vi "Reset All CMDS.vi"(8 "error in (no error)":errorcluster) -> (0 "error out":errorcluster)   [LabVIEW 2018]
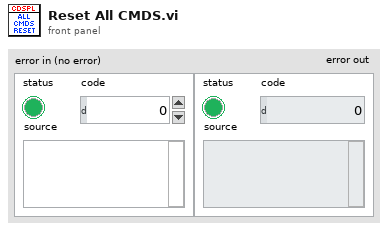
[diagram p1: front panel]
types:
  T1 = enum16{"Lamp A1", "Lamp B1", "Lamp C1", "Lamp D1", "Lamp E1", "Lamp F1", "Lamp G1", "Lamp H1", "Lamp A2", "Lamp B2", "Lamp C2", "Lamp D2", "Lamp E2", "Lamp F2", "Lamp G2", "Lamp H2", "Ack A1", "Ack B1", "Ack C1", "Ack D1", "Ack E1", "Ack F1", "Ack G1", "Ack H1", "Ack A2", "Ack B2", "Ack C2", "Ack D2", "Ack E2", "Ack F2", "Ack G2", "Ack H2", "SSM", "SAS", "LSM", ""}
  T2 = enum16{"Lamp A1", "Lamp B1", "Lamp C1", "Lamp D1", "Lamp E1", "Lamp F1", "Lamp G1", "Lamp H1", "Lamp A2", "Lamp B2", "Lamp C2", "Lamp D2", "Lamp E2", "Lamp F2", "Lamp G2", "Lamp H2", "Ack A1", "Ack B1", "Ack C1", "Ack D1", "Ack E1", "Ack F1", "Ack G1", "Ack H1", "Ack A2", "Ack B2", "Ack C2", "Ack D2", "Ack E2", "Ack F2", "Ack G2", "Ack H2", "SSM", "SAS", "LSM", ""}[]
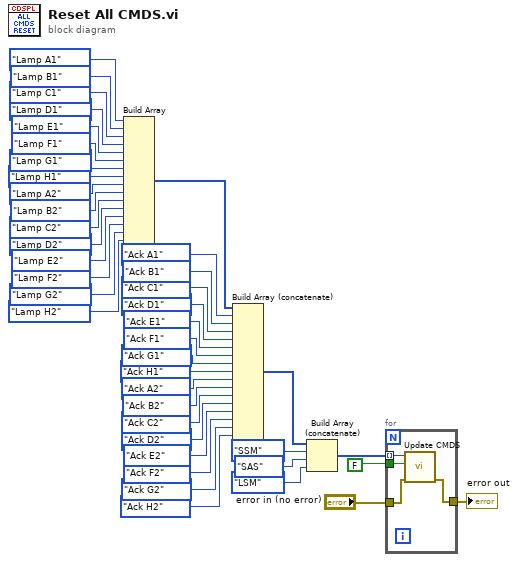
[diagram p0: block diagram]
diagram:
  n1 = Build Array(T1."Lamp A1" ("Tag"), T1."Lamp B1" ("Tag"), T1."Lamp C1" ("Tag"), T1."Lamp D1" ("Tag"), T1."Lamp E1" ("Tag"), T1."Lamp F1" ("Tag"), T1."Lamp G1" ("Tag"), T1."Lamp H1" ("Tag"), T1."Lamp A2" ("Tag"), T1."Lamp B2" ("Tag"), T1."Lamp C2" ("Tag"), T1."Lamp D2" ("Tag"), T1."Lamp E2" ("Tag"), T1."Lamp F2" ("Tag"), T1."Lamp G2" ("Tag"), T1."Lamp H2" ("Tag")) -> (w8:T2)
  n2 = Build Array (concatenate)(w8, T1."Ack A1" ("Tag"), T1."Ack B1" ("Tag"), T1."Ack C1" ("Tag"), T1."Ack D1" ("Tag"), T1."Ack E1" ("Tag"), T1."Ack F1" ("Tag"), T1."Ack G1" ("Tag"), T1."Ack H1" ("Tag"), T1."Ack A2" ("Tag"), T1."Ack B2" ("Tag"), T1."Ack C2" ("Tag"), T1."Ack D2" ("Tag"), T1."Ack E2" ("Tag"), T1."Ack F2" ("Tag"), T1."Ack G2" ("Tag"), T1."Ack H2" ("Tag")) -> (w7:T2)
  n3 = Build Array (concatenate)(w7, T1."SSM" ("Tag"), T1."SAS" ("Tag"), T1."LSM" ("Tag")) -> (w3:T2)
  n4 = for {
    tunnel: FALSE ("Value") -> [w45]
    tunnel: w3 -> [w44] mode=indexing
    tunnel: "error in (no error)" -> [w43]
    tunnel: [w42] -> w1
    n5 = call "Update CMDS.vi"("error in (no error)"=w43, "New Value"=w45, "Tag"=w44) -> ("error out"=w42:errorcluster)  [unwired: 8 in]
  }
  "error out" <- w1
